vi "Read Return Header.vi"(8 "error in (no error)":errorcluster, 10 "Name":string, 11 "WebSocket in":refnum<class "WebSocket.lvclass">) -> (0 "error out":errorcluster, 1 "Found?":bool, 2 "Value":string, 3 "WebSocket out":refnum<class "WebSocket.lvclass">)   [LabVIEW 2013, in "WebSockets.lvlib" / "WebSocket.lvclass"]
doc: "Retrieves a named header from the received HTTP handshaking data."
uses:
  WebSocket.lvclass
  WebSocket.lvclass/WebSocket.ctl
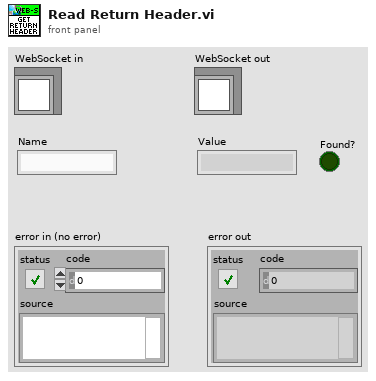
[diagram p1: front panel]
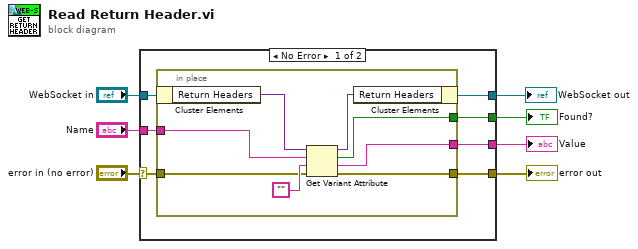
[diagram p0: block diagram]
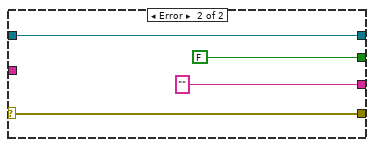
[diagram p2: hidden frame]
diagram:
  n1 = case shown="No Error" "error in (no error)" {
    selector: "error in (no error)" -> [w12 w26]
    tunnel: [w14 ""] -> w7
    tunnel: "Name" -> [w13 _]
    tunnel: "WebSocket in" -> [w9 w25]
    tunnel: [w8 w25] -> w2
    tunnel: [w11 w26] -> w4
    tunnel: [w10 FALSE] -> w3
    frame No Error {
      n2 = in-place {
        in-place-border: [w22] -> w14
        in-place-border: w13 -> [w20]
        in-place-border: w12 -> [w19]
        in-place-border: [w18] -> w11
        in-place-border: [w17] -> w10
        n3 = in-place-cluster #1(w9) -> ("Return Headers"=w16:variant)
        n4 = Get Variant Attribute(Variant=w16, name=w20, default value (empty Variant)="", error in=w19) -> (duplicate Variant=w15:variant, found=w17:bool, value=w22:string, error out=w18:errorcluster)
        n5 = in-place-cluster #1("Return Headers"=w15) -> (w8:refnum<class "WebSocket.lvclass">)
      }
    }
    frame Error {
    }
  }
  "Value" <- w7
  "error out" <- w4
  "Found?" <- w3
  "WebSocket out" <- w2
